vi "Initialize Test.vi"(11 "Executioner in":refnum<class "Executioner.lvclass">) -> (3 "Executioner out":refnum<class "Executioner.lvclass">)   [LabVIEW 2019, in "Test Executive.lvlib" / "Executioner.lvclass"]
uses:
  <vilib>/gpm_packages/@cs/test-executive/Source/Test Executive/Executioner/Executioner.lvclass
  <vilib>/gpm_packages/@cs/test-executive/Source/Test Executive/Executioner/Executioner.lvclass/Executioner.ctl
  <vilib>/gpm_packages/@cs/lookup-table/Source/LookupTable/LookupTable.lvclass
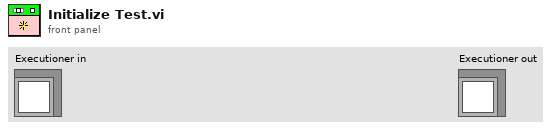
[diagram p1: front panel]
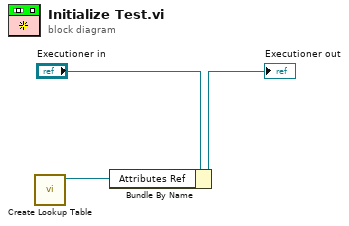
[diagram p0: block diagram]
diagram:
  n1 = call <vilib>:"Create Lookup Table.vi"() -> ("LookupTable Reference"=w1:refnum<data-value>)  [unwired: 10 in, 1 out]
  n2 = Bundle By Name(cluster="Executioner in", "Attributes Ref"=w1) -> (→"Executioner out":refnum<class "Executioner.lvclass">)
